vi "Qudi_ROI_multicolour_scan.vi"(3 "N Z positions":i32) -> ()   [LabVIEW 2015]
uses:
  <vilib>/rvi/Analysis/control/PID/Typedef/niFpgaPID_PIGains.ctl
  <vilib>/Platform/TimedLoop/XDataNode/timing_clust.ctl
  <vilib>/Platform/TimedLoop/XDataNode/nitl_modes.ctl
  <vilib>/Platform/TimedLoop/XDataNode/wakeup.ctl
  <vilib>/rvi/FXPMathLib/basic elements/FxpIntAccumulator/subVIs/nifxpmath_IntAccumulator_SimConfig.ctl
  <vilib>/rvi/Emulation/niFpgaGetClockAttributes.vi
  <vilib>/rvi/Emulation/niFpgaSctlEmulationGetInTimedLoop.vi
  <vilib>/rvi/Emulation/niFpgaEmulationReportErrorSimple.vi
  <vilib>/rvi/Emulation/niFpgaProcessEmulError.vi
  <vilib>/rvi/eio/common/nirviEmuTemplateMethod_errors.vi
  <vilib>/rvi/Analysis/common/codeGenErrors/XNode/niFpgaXNodeCodeGenErrorHandle.vi
  <vilib>/rvi/Emulation/niFpgaCriticalErrorInLSC.vi
  <vilib>/rvi/FXPMathLib/basic elements/FxpIntAccumulator/simVIs/DllFxpIntAccumulator_sub.vi
  <vilib>/rvi/Analysis/control/PID/SubVIs/niFpgaPID_PIWrapper.vi
  <vilib>/eio/EIONode/EIONode.xnode
  <vilib>/rvi/Analysis/measure/dc-rms/XNode/niFpgaDC-RMS.xnode
  <vilib>/Platform/TimedLoop/XDataNode/XDataNode.xnode
  <vilib>/rvi/FXPMathLib/basic elements/FxpIntAccumulator/XNode/nifxpmath_IntAccumulator.xnode
  <vilib>/rvi/FXPMathLib/FxpMul/XNode/nifxpmath_Multiplier.xnode
  <vilib>/Platform/TimedLoop/XDataNode/XDNodeRunTimeDep.lvlib
  <vilib>/rvi/FXPMathLib/sim/FxpSim.dll
panel:
  out "duration_ms":u32
  out "X":i16
  out "Y":i16
  out "Sum":i16
  out "counter":u32
  out "output":i16
  in  "reset":bool
  in  "reset_counter":bool
  in  "autofocus":bool
  in  "setpoint":i16
  in  "P":i16
  in  "I":i16
  in  "ref_axis":bool
  in  "integration_time_us":u32=100 caption="Count(uSec)"
  in  "exposure_time_ms":u16
  in  "stop":bool
  out "n cycles":i32
  out "Images acquired":i32
  in  "Laser lines":i32[](array[numeric])=[0, 0, 0, 0, 0, 0, 0, 0, 0, 0]
  in  "N laser lines":i32
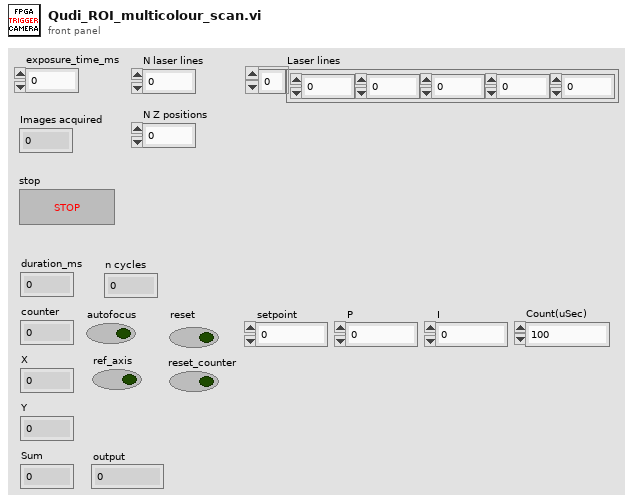
[diagram p1: front panel]
types:
  T1 = typedef "niFpgaPID_PIGains.ctl" = cluster{"proportional gain":sgl, "integral gain":sgl}
  T2 = typedef "XDNodeRunTimeDep.lvlib/timing_clust.ctl" = cluster{"Expected End [f-1]":u64, "Actual End [f-1]":u64, "Finished Late? [f-1]":bool, "Expected End [i-1]":u64, "Actual End [i-1]":u64, "Finished Late? [i-1]":bool, "Expected Start [i]":u64, "Actual Start [i]":u64, "Expected Start [f]":u64, "Actual Start [f]":u64, "Source Name":string, "Structure Name":string, "Period":i64, "Deadline":i64, "Offset":i64, "Start":i64, "Priority":i32, "Timeout":i32, "Mode":T3, "Wakeup Reason":T4, "Error":errorcluster, "Source Type":string, "Secondary Source Type":string, "Global End Time":u64, "Global Start Time":u64, "Frame Duration":u64, "Iteration Duration":u64, "Assigned CPU":i32, "I/O Scan Engine Mode":u32}
  T3 = typedef "XDNodeRunTimeDep.lvlib/nitl_modes.ctl" = enum32{"No Change", "Process missed periods, maintain original phase", "Discard missed periods, maintain original phase", "Process missed periods, ignore original phase", "Discard missed periods, ignore original phase"}
  T4 = typedef "XDNodeRunTimeDep.lvlib/wakeup.ctl" = enum32{"Normal", "Aborted", "Asynchronous wakeup", "Timing source error", "Timed loop error", "Timeout"}
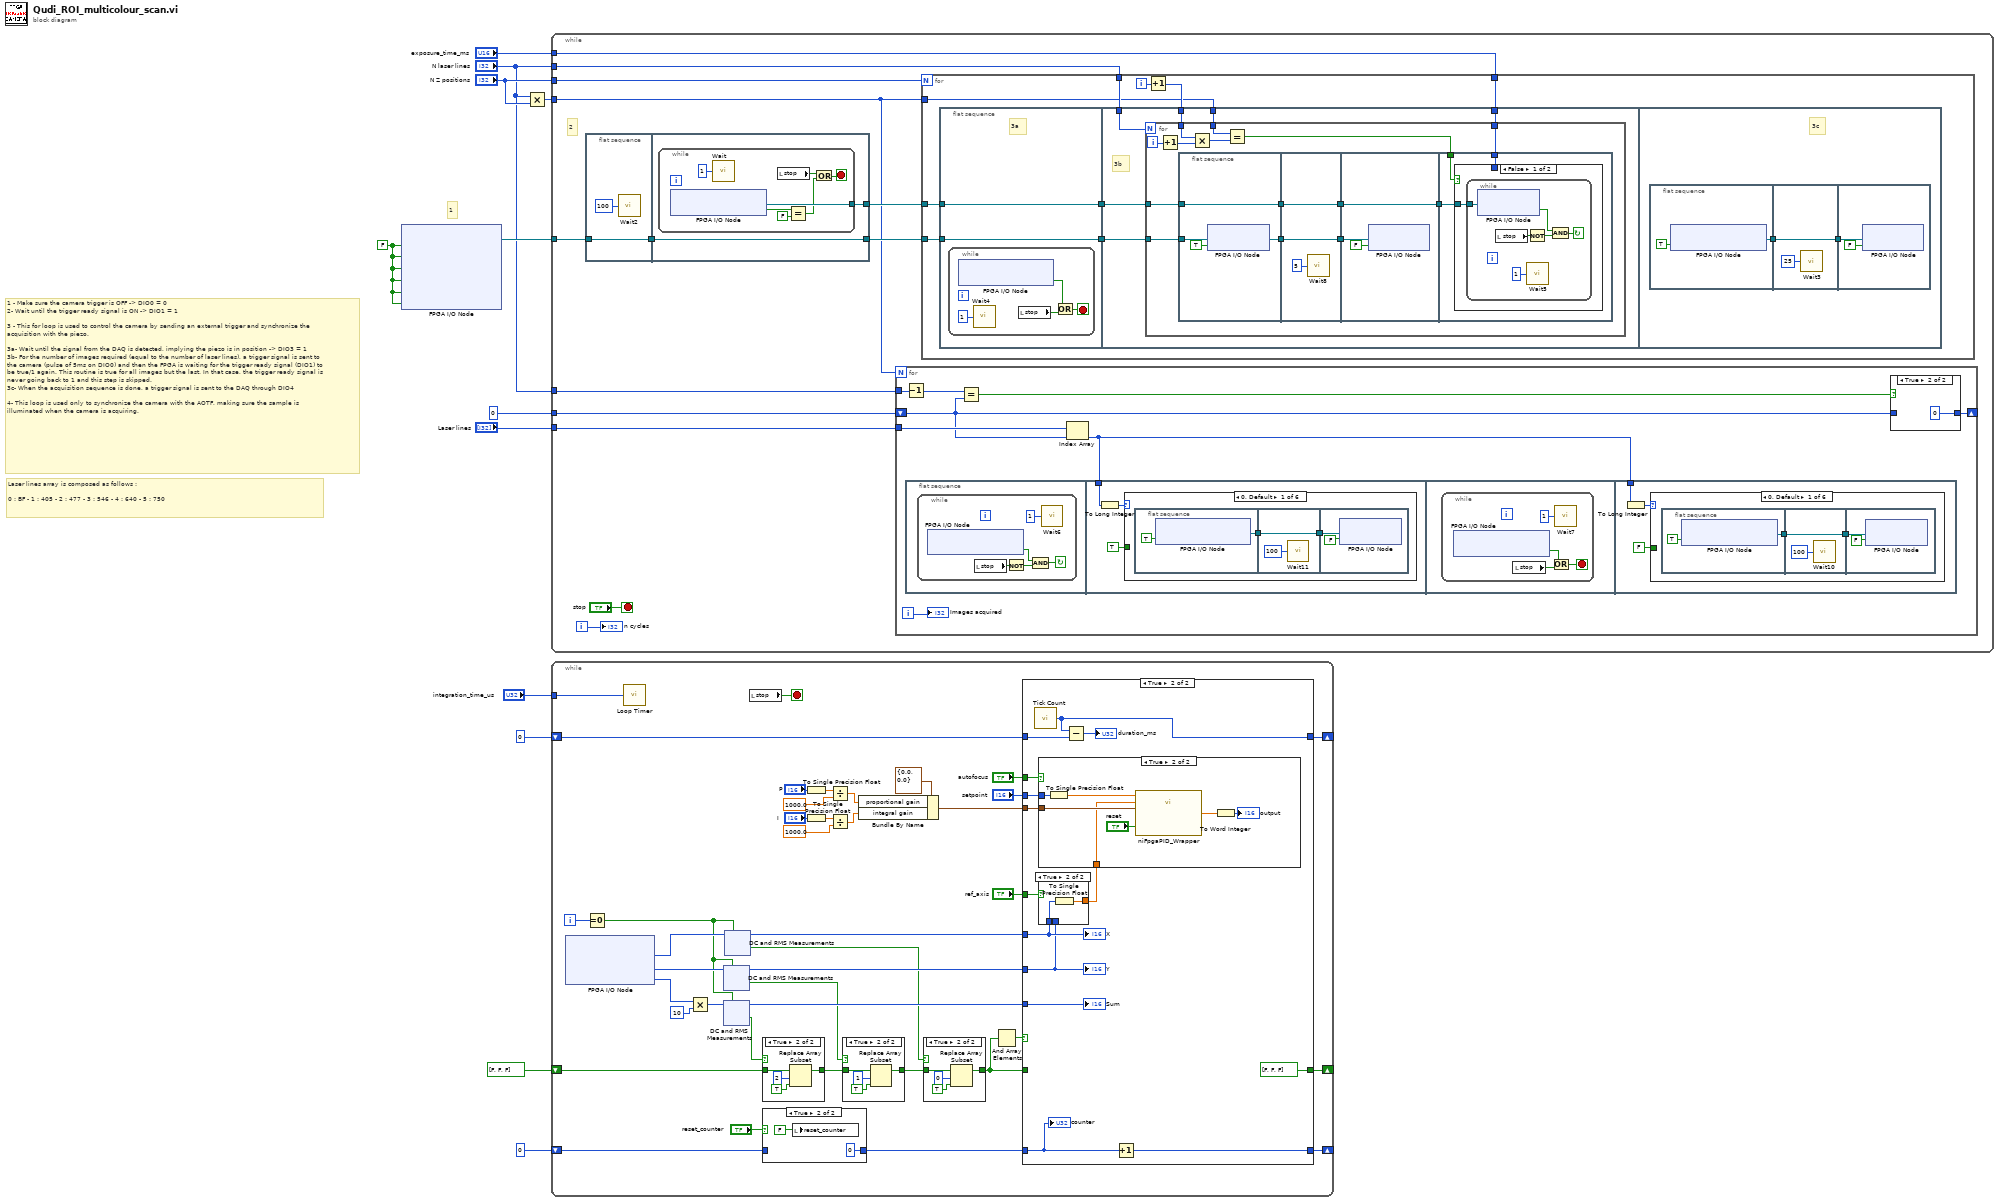
[diagram p0: block diagram]
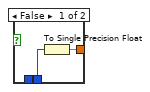
[diagram p7: hidden frame]
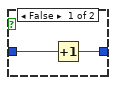
[diagram p9: hidden frame]
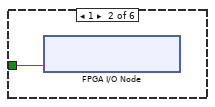
[diagram p10: hidden frame]
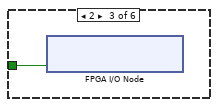
[diagram p11: hidden frame]
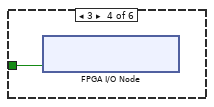
[diagram p12: hidden frame]
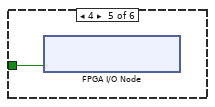
[diagram p13: hidden frame]
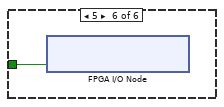
[diagram p14: hidden frame]
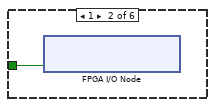
[diagram p15: hidden frame]
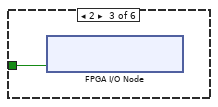
[diagram p16: hidden frame]
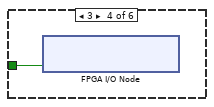
[diagram p17: hidden frame]
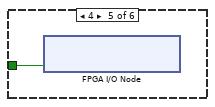
[diagram p18: hidden frame]
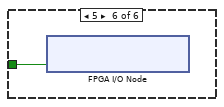
[diagram p19: hidden frame]
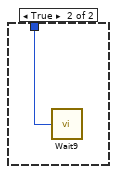
[diagram p20: hidden frame]
diagram:
  w5 = FALSE ("Connector0/DIO0")
  # "Laser lines array is composed as follows :\n\n0 : BF - 1 : 405 - 2 : 477 - 3 : 546 - 4 : 640 - 5 : 750"
  # "1"
  # "1 - Make sure the camera trigger is OFF -> DIO0 = 0\n2- Wait until the trigger ready signal is ON -> DIO1 = 1\n\n3 - This for loop is used to control the camera by sending an external trigger and synchronize the acquisition with the piezo.\n\n3a- Wait until the signal from the DAQ is detected, implying the piezo is in position -> DIO3 = 1 \n3b- For the number of images required (equal to the number of laser lines), a trigger signal is sent to the camera (pulse of 5ms on DIO0) and then the FPGA is waiting for the trigger ready signal (DIO1) to be true/1 again. This routine is true for all images but the last. In that case, the trigger ready signal is never going back to 1 and this step is skipped. \n3c- When the acquisition sequence is done, a trigger signal is sent to the DAQ through DIO4\n\n4- This loop is used only to synchronize the camera with the AOTF, making sure the sample is illuminated when the camera is acquiring."
  n1 = xnode "FPGA I/O Node"("Connector0/DIO0"=w5, "Connector0/DIO6"=w5, "Connector0/DIO7"=w5, "Connector0/DIO8"=w5, "Connector0/DIO9"=w5, "Connector0/DIO10"=w5) -> ("FPGA I/O Out"=w12:refnum<k21>)  [unwired: 6 in, 5 out]
  n2 = Multiply(x="N laser lines", y="N Z positions") -> (x*y=w8:i32)
  n3 = while {
    tunnel: w12 -> [w24]
    tunnel: "Laser lines" -> [w21]
    tunnel: 0 -> [w20]
    tunnel: "N Z positions" -> [w19]
    tunnel: "N laser lines" -> [w17]
    tunnel: w8 -> [w16]
    tunnel: "N laser lines" -> [w15]
    tunnel: "exposure_time_ms" -> [w14]
    i -> [w18]
    stop <- "stop" stop-if-true
    # "2"
    n4 = flat-sequence {
      tunnel: w24 -> [w79]
      tunnel: [w79] -> w25
      tunnel: w25 -> [w81]
      tunnel: [w81] -> w23
      tunnel: [w80] -> w22
      frame #0 {
        n5 = call "Wait2"("Count(uSec)"=u8 100 ("Count(mSec)")) -> ()  [unwired: 1 out]
      }
      frame #1 {
        n6 = while {
          tunnel: [w88] -> w80
          stop <- w83 stop-if-true
          n7 = xnode "FPGA I/O Node"() -> ("Connector0/DIO1"=w87:bool, "FPGA I/O Out"=w88:refnum<k21>)  [unwired: 1 in]
          n8 = call "Wait"("Count(mSec)"=u8 1) -> ()  [unwired: 1 out]
          n9 = local read "stop"() -> (w84:bool)
          n10 = Equal?(x=w87, y=FALSE) -> (x = y?=w85:bool)
          n11 = Or(x=w84, y=w85) -> (x .or. y?=w83:bool)
        }
      }
    }
    n12 = for {
      N: w16 -> [_]
      shift-right: [w31] -> _
      shift-left: w20 -> [w29]
      tunnel: w21 -> [w30]
      tunnel: w15 -> [w28]
      i -> [w26]
      n13 = Decrement(x=w28) -> (x-1=w27:i32)
      n14 = flat-sequence {
        tunnel: w33 -> [w43]
        tunnel: w33 -> [w62]
        frame #0 {
          n15 = while {
            stop <- w38 continue-if-true
            n16 = xnode "FPGA I/O Node"() -> ("Connector0/DIO2"=w39:bool)  [unwired: 1 in, 1 out]
            n17 = local read "stop"() -> (w40:bool)
            n18 = Not(x=w40) -> (.not. x?=w41:bool)
            n19 = And(x=w39, y=w41) -> (x .and. y?=w38:bool)
            n20 = call "Wait6"("Count(mSec)"=u8 1) -> ()  [unwired: 1 out]
          }
        }
        frame #1 {
          n21 = To Long Integer(number=w43) -> (32bit integer=w44:i32)
          n22 = case shown="0, Default" w44 {
            tunnel: TRUE ("Connector0/DIO6") -> [_ w53 w54 w55 w56 w57]
            frame 0, Default {
              n23 = flat-sequence {
                tunnel: [w47] -> w46
                tunnel: w46 -> [w49]
                tunnel: [w49] -> w45
                tunnel: w45 -> [w52]
                frame #0 {
                  n24 = xnode "FPGA I/O Node"("Connector0/DIO5"=TRUE) -> ("FPGA I/O Out"=w47:refnum<k21>)  [unwired: 1 in]
                }
                frame #1 {
                  n25 = call "Wait11"("Count(uSec)"=u32 100) -> ()  [unwired: 1 out]
                }
                frame #2 {
                  n26 = xnode "FPGA I/O Node"("I/O Item"=FALSE, "FPGA I/O In"=w52) -> ()  [unwired: 1 out]
                }
              }
            }
            frame 1 {
              n27 = xnode "FPGA I/O Node"("Connector0/DIO8"=w53) -> ()  [unwired: 1 in, 1 out]
            }
            frame 2 {
              n28 = xnode "FPGA I/O Node"("Connector0/DIO9"=w54) -> ()  [unwired: 1 in, 1 out]
            }
            frame 3 {
              n29 = xnode "FPGA I/O Node"("Connector0/DIO6"=w55) -> ()  [unwired: 1 in, 1 out]
            }
            frame 4 {
              n30 = xnode "FPGA I/O Node"("Connector0/DIO7"=w56) -> ()  [unwired: 1 in, 1 out]
            }
            frame 5 {
              n31 = xnode "FPGA I/O Node"("Connector0/DIO10"=w57) -> ()  [unwired: 1 in, 1 out]
            }
          }
        }
        frame #2 {
          n32 = while {
            stop <- w59 stop-if-true
            n33 = xnode "FPGA I/O Node"() -> ("Connector0/DIO2"=w60:bool)  [unwired: 1 in, 1 out]
            n34 = local read "stop"() -> (w61:bool)
            n35 = Or(x=w60, y=w61) -> (x .or. y?=w59:bool)
            n36 = call "Wait7"("Count(mSec)"=u8 1) -> ()  [unwired: 1 out]
          }
        }
        frame #3 {
          n37 = To Long Integer(number=w62) -> (32bit integer=w63:i32)
          n38 = case shown="0, Default" w63 {
            tunnel: FALSE ("Connector0/DIO6") -> [_ w73 w74 w75 w76 w77]
            frame 0, Default {
              n39 = flat-sequence {
                tunnel: [w67] -> w66
                tunnel: w66 -> [w69]
                tunnel: [w69] -> w65
                tunnel: w65 -> [w72]
                frame #0 {
                  n40 = xnode "FPGA I/O Node"("Connector0/DIO5"=TRUE) -> ("FPGA I/O Out"=w67:refnum<k21>)  [unwired: 1 in]
                }
                frame #1 {
                  n41 = call "Wait10"("Count(uSec)"=u32 100) -> ()  [unwired: 1 out]
                }
                frame #2 {
                  n42 = xnode "FPGA I/O Node"("I/O Item"=FALSE, "FPGA I/O In"=w72) -> ()  [unwired: 1 out]
                }
              }
            }
            frame 1 {
              n43 = xnode "FPGA I/O Node"("Connector0/DIO8"=w73) -> ()  [unwired: 1 in, 1 out]
            }
            frame 2 {
              n44 = xnode "FPGA I/O Node"("Connector0/DIO9"=w74) -> ()  [unwired: 1 in, 1 out]
            }
            frame 3 {
              n45 = xnode "FPGA I/O Node"("Connector0/DIO6"=w75) -> ()  [unwired: 1 in, 1 out]
            }
            frame 4 {
              n46 = xnode "FPGA I/O Node"("Connector0/DIO7"=w76) -> ()  [unwired: 1 in, 1 out]
            }
            frame 5 {
              n47 = xnode "FPGA I/O Node"("Connector0/DIO10"=w77) -> ()  [unwired: 1 in, 1 out]
            }
          }
        }
      }
      n48 = Equal?(x=w27, y=w29) -> (x = y?=w32:bool)
      n49 = Index Array(array=w30, index=w29) -> (element=w33:i32)
      n50 = case shown="True" w32 {
        tunnel: w29 -> [w35 _]
        tunnel: [w34 0] -> w31
        frame False {
          n51 = Increment(x=w35) -> (x+1=w34:i32)
        }
        frame True {
        }
      }
      "Images acquired" <- w26
    }
    n52 = for {
      N: w19 -> [_]
      tunnel: w23 -> [w96]
      tunnel: w22 -> [w97]
      tunnel: w17 -> [w92]
      tunnel: w16 -> [w90]
      tunnel: w14 -> [w89]
      i -> [w93]
      n53 = flat-sequence {
        tunnel: w96 -> [w98]
        tunnel: w97 -> [w99]
        tunnel: [w99] -> w95
        tunnel: [w98] -> w94
        tunnel: w95 -> [w109]
        tunnel: w94 -> [w108]
        tunnel: w92 -> [w107]
        tunnel: w91 -> [w106]
        tunnel: w90 -> [w105]
        tunnel: w89 -> [w104]
        frame #0 {
          # "3a"
          n54 = while {
            stop <- w101 stop-if-true
            n55 = xnode "FPGA I/O Node"() -> ("Connector0/DIO3"=w102:bool)  [unwired: 1 in, 1 out]
            n56 = call "Wait4"("Count(mSec)"=u8 1) -> ()  [unwired: 1 out]
            n57 = local read "stop"() -> (w103:bool)
            n58 = Or(x=w102, y=w103) -> (x .or. y?=w101:bool)
          }
        }
        frame #1 {
          # "3b"
          n59 = for {
            N: w107 -> [_]
            tunnel: w109 -> [w118]
            tunnel: w108 -> [w117]
            tunnel: w106 -> [w114]
            tunnel: w105 -> [w112]
            tunnel: w104 -> [w110]
            i -> [w116]
            n60 = Increment(x=w116) -> (x+1=w115:i32)
            n61 = flat-sequence {
              tunnel: [w126] -> w123
              tunnel: [w124] -> w122
              tunnel: w117 -> [w125]
              tunnel: w118 -> [w124]
              tunnel: w123 -> [w130]
              tunnel: [w130] -> w121
              tunnel: [w129] -> w120
              tunnel: w122 -> [w129]
              tunnel: w121 -> [w132]
              tunnel: [w131] -> w119
              tunnel: w120 -> [w131]
              tunnel: w119 -> [w136]
              tunnel: w111 -> [w135]
              tunnel: w110 -> [w134]
              frame #0 {
                n62 = xnode "FPGA I/O Node"("I/O Item"=TRUE ("Connector0/DIO0"), "FPGA I/O In"=w125) -> ("FPGA I/O Out"=w126:refnum<k21>)
              }
              frame #1 {
                n63 = call "Wait8"("Count(mSec)"=u8 5) -> ()  [unwired: 1 out]
              }
              frame #2 {
                n64 = xnode "FPGA I/O Node"("I/O Item"=FALSE ("Connector0/DIO0"), "FPGA I/O In"=w132) -> ()  [unwired: 1 out]
              }
              frame #3 {
                n65 = case shown="False" w135 {
                  tunnel: w136 -> [w137 _]
                  tunnel: w134 -> [_ w144]
                  frame False {
                    n66 = while {
                      tunnel: w137 -> [w143]
                      stop <- w139 continue-if-true
                      n67 = xnode "FPGA I/O Node"("FPGA I/O In"=w143) -> ("I/O Item"=w140:bool)  [unwired: 1 out]
                      n68 = local read "stop"() -> (w142:bool)
                      n69 = Not(x=w142) -> (.not. x?=w141:bool)
                      n70 = call "Wait5"("Count(mSec)"=u8 1) -> ()  [unwired: 1 out]
                      n71 = And(x=w140, y=w141) -> (x .and. y?=w139:bool)
                    }
                  }
                  frame True {
                    n72 = call "Wait9"("Count(mSec)"=w144) -> ()  [unwired: 1 out]
                  }
                }
              }
            }
            n73 = Multiply(x=w114, y=w115) -> (x*y=w113:i32)
            n74 = Equal?(x=w112, y=w113) -> (x = y?=w111:bool)
          }
        }
        frame #2 {
          # "3c"
          n75 = flat-sequence {
            tunnel: [w148] -> w146
            tunnel: w146 -> [w149]
            tunnel: [w149] -> w145
            tunnel: w145 -> [w151]
            frame #0 {
              n76 = xnode "FPGA I/O Node"("Connector0/DIO4"=TRUE) -> ("FPGA I/O Out"=w148:refnum<k21>)  [unwired: 1 in]
            }
            frame #1 {
              n77 = call "Wait3"("Count(mSec)"=u8 25) -> ()  [unwired: 1 out]
            }
            frame #2 {
              n78 = xnode "FPGA I/O Node"("I/O Item"=FALSE ("Connector0/DIO0"), "FPGA I/O In"=w151) -> ()  [unwired: 1 out]
            }
          }
        }
      }
      n79 = Increment(x=w93) -> (x+1=w91:i32)
    }
    "n cycles" <- w18
  }
  n80 = while {
    shift-right: [w177] -> _
    shift-left: bool[] [FALSE, FALSE, FALSE] ("initialized array") -> [w185]
    shift-right: [w175] -> _
    shift-left: u32 0 -> [w176]
    tunnel: "integration_time_us" -> [w174]
    shift-right: [w173] -> _
    shift-left: u32 0 -> [w171]
    i -> [w191]
    stop <- w153 stop-if-true
    n81 = xnode "FPGA I/O Node"() -> ("Connector0/AI0"=w192:i16, "Connector0/AI1"=w189:i16, "Connector0/AI2"=w156:i16)  [unwired: 3 in, 3 out]
    n82 = Equal To 0?(x=w191) -> (x = 0?=w186:bool)
    n83 = call "Loop Timer"("Count(uSec)"=w174) -> ()  [unwired: 1 out]
    n84 = Multiply(x=w156, y=i16 10) -> (x*y=w155:i16)
    n85 = xnode "DC and RMS Measurements"("input data"=w189, "reset"=w186) -> ("DC"=w188:i16, "output valid"=w181:bool)
    n86 = xnode "DC and RMS Measurements"("input data"=w155, "reset"=w186) -> ("DC"=w187:i16, "output valid"=w182:bool)
    n87 = xnode "DC and RMS Measurements"("input data"=w192, "reset"=w186) -> ("DC"=w190:i16, "output valid"=w180:bool)
    n88 = local read "stop"() -> (w153:bool)
    n89 = case shown="True" w182 {
      tunnel: w185 -> [w201 w204]
      tunnel: [w201 w202] -> w184
      frame False {
      }
      frame True {
        n90 = Replace Array Subset(array=w204, new element=TRUE, index=2) -> (w202:bool[])
      }
    }
    n91 = case shown="True" "reset_counter" {
      tunnel: w171 -> [w193 _]
      tunnel: [w193 u32 0] -> w170
      frame False {
      }
      frame True {
        n92 = local write "reset_counter"(FALSE ("Reset counter")) -> ()
      }
    }
    n93 = To Single Precision Float(number="P") -> (single precision float=w163:sgl)
    n94 = To Single Precision Float(number="I") -> (single precision float=w160:sgl)
    n95 = Divide(x=w163, y=sgl 1000.0) -> (x/y=w161:sgl)
    n96 = Divide(x=w160, y=sgl 1000.0) -> (x/y=w158:sgl)
    n97 = case shown="True" w181 {
      tunnel: w184 -> [w206 w209]
      tunnel: [w206 w207] -> w183
      frame False {
      }
      frame True {
        n98 = Replace Array Subset(array=w209, new element=TRUE, index=1) -> (w207:bool[])
      }
    }
    n99 = Bundle By Name(cluster=T1 {"proportional gain"=0.0, "integral gain"=0.0} ("gains"), "proportional gain"=w161, "integral gain"=w158) -> (w164:T1)
    n100 = case shown="True" w180 {
      tunnel: [w196 w198] -> w178
      tunnel: w183 -> [w196 w197]
      frame False {
      }
      frame True {
        n101 = Replace Array Subset(array=w197, new element=TRUE, index=0) -> (w198:bool[])
      }
    }
    n102 = And Array Elements(Boolean array=w178) -> (logical AND=w179:bool)
    n103 = case shown="True" w179 {
      tunnel: w190 -> [_ w216]
      tunnel: w188 -> [_ w214]
      tunnel: w187 -> [_ w222]
      tunnel: w178 -> [w213 _]
      tunnel: [w213 bool[] [FALSE, FALSE, FALSE] ("initialized array")] -> w177
      tunnel: w176 -> [w212 w226]
      tunnel: [w212 w224] -> w175
      tunnel: w170 -> [w211 w221]
      tunnel: [w211 w223] -> w173
      tunnel: "autofocus" -> [_ w220]
      tunnel: "setpoint" -> [_ w219]
      tunnel: w164 -> [_ w218]
      tunnel: "ref_axis" -> [_ w217]
      frame False {
      }
      frame True {
        n104 = call "Tick Count"() -> ("Tick Count(mSec)"=w224:u32)
        n105 = case shown="True" w217 {
          tunnel: w216 -> [_ w231]
          tunnel: [w228 w230] -> w215
          tunnel: w214 -> [w229 _]
          frame False {
            n106 = To Single Precision Float(number=w229) -> (single precision float=w228:sgl)
          }
          frame True {
            n107 = To Single Precision Float(number=w231) -> (single precision float=w230:sgl)
          }
        }
        n108 = case shown="True" w220 {
          tunnel: w219 -> [_ w238]
          tunnel: w218 -> [_ w236]
          tunnel: w215 -> [_ w232]
          frame False {
          }
          frame True {
            n109 = To Single Precision Float(number=w238) -> (single precision float=w237:sgl)
            n110 = call-poly <vilib>:"niFpgaPID_Wrapper.vi"("setpoint"=w237, "reset? (F)"="reset", "process variable"=w232, "gains"=w236) -> ("output"=w234:sgl)  [unwired: 9 in, 2 out]
            n111 = To Word Integer(number=w234) -> (16bit integer=→"output":i16)
          }
        }
        n112 = Subtract(x=w224, y=w226) -> (x-y=→"duration_ms":u32)
        n113 = Increment(x=w221) -> (x+1=w223:u32)
        "X" <- w216
        "Y" <- w214
        "Sum" <- w222
        "counter" <- w221
      }
    }
  }
